vi "mph_to_mps.vi"(1 "Miles/hour":sgl format="%.3g") -> (0 "Meter/second":sgl format="%.3f")   [LabVIEW 2012]
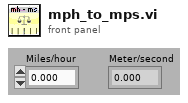
[diagram p1: front panel]
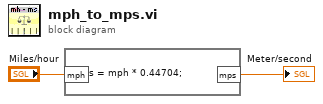
[diagram p0: block diagram]
diagram:
  n1 = formula code="mps = mph * 0.44704;"("mph"="Miles/hour") -> ("mps"=→"Meter/second":dbl)
